vi "NodesToAbsCoordinates.vi"(8 "error in":errorcluster, 9 "Coordinates":cluster{"X":dbl, "Y":dbl}[](array[cluster]), 10 "Path":i32[](array[numeric])) -> (0 "error out":errorcluster, 2 "Points output":T1)   [LabVIEW 2009, in "Main.lvlib"]
uses:
  Main.lvlib
  Navigation/Nav_CordinateArray.ctl
  Navigation.lvlib
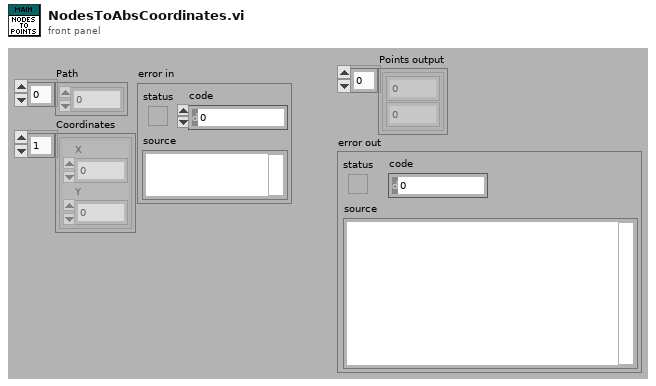
[diagram p1: front panel]
types:
  T1 = typedef "Navigation.lvlib/Nav_CordinateArray.ctl" = cluster{"X position":dbl, "Y position":dbl}[]
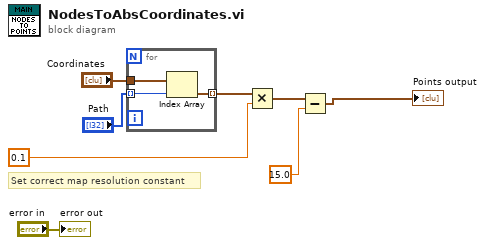
[diagram p0: block diagram]
diagram:
  # "Set correct map resolution constant"
  n1 = for {
    tunnel: "Coordinates" -> [w11]
    tunnel: "Path" -> [w10] mode=indexing
    tunnel: [w9] -> w6 mode=indexing
    n2 = Index Array(array=w11, index=w10) -> (element=w9:cluster{"X":dbl, "Y":dbl})
  }
  n3 = Multiply(x=w6, y=0.1 ("X")) -> (x*y=w3:cluster{"X":dbl, "Y":dbl}[])
  n4 = Subtract(x=w3, y=15.0 ("X")) -> (x-y=→"Points output":cluster{"X":dbl, "Y":dbl}[])
  "error out" <- "error in"
